vi "Undo.vi"(8 "error in (no error)":errorcluster, 11 "All Queue in":T2) -> (0 "error out":errorcluster, 2 "Ctrl Val.Get All":T1[](array[typedef]), 3 "All Queue out":T2, 4 "Redo Enable":bool, 6 "Undo Enable":bool)   [LabVIEW 2015, in "UndoLibrary.lvlib"]
doc: "This VI stores the values to perform the undo action."
uses:
  UndoLibrary.lvlib
  Controls/cluster_All Queue.ctl
  Controls/cluster_Control Value.ctl
  QueueOperations/QueueOperations.lvlib
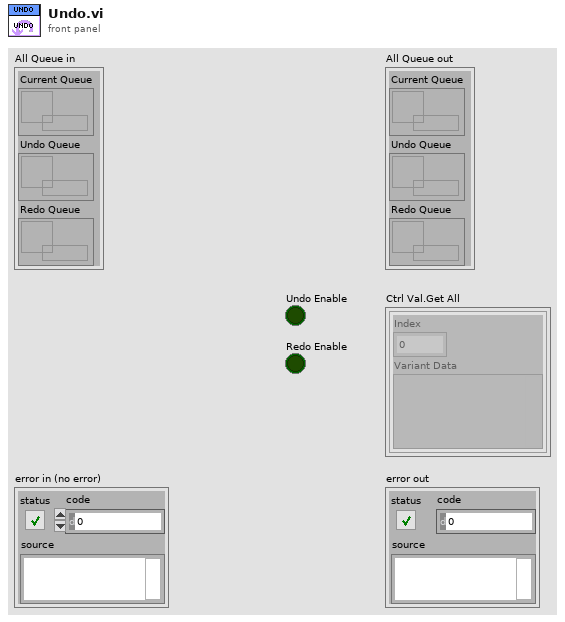
[diagram p1: front panel]
types:
  T1 = typedef "UndoLibrary.lvlib/cluster_Control Value.ctl" = cluster{"Index":i32, "Variant Data":variant}
  T2 = typedef "UndoLibrary.lvlib/cluster_All Queue.ctl" = cluster{"Current Queue":refnum<queue>, "Undo Queue":refnum<queue>, "Redo Queue":refnum<queue>}
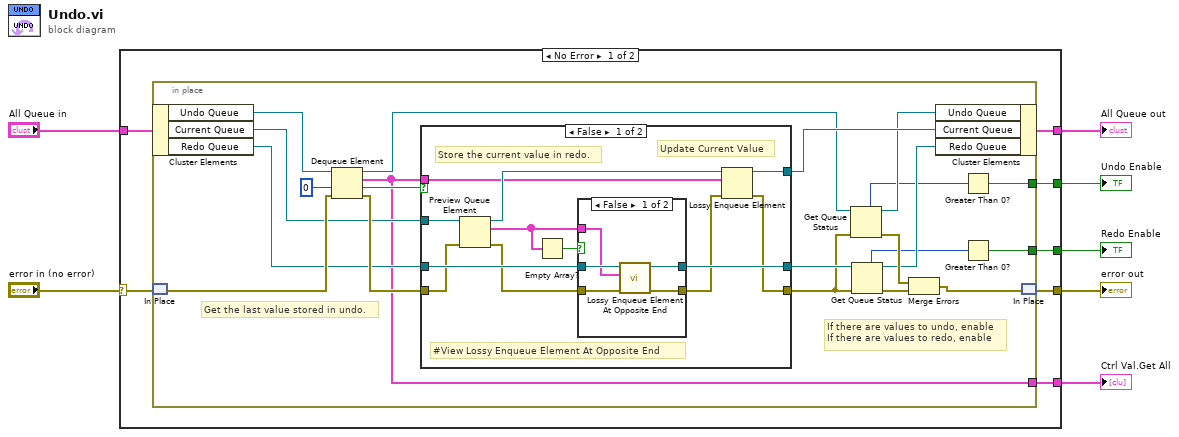
[diagram p0: block diagram]
diagram:
  n1 = case shown="No Error" "error in (no error)" {
    selector: "error in (no error)" -> [w14 w59]
    tunnel: [w13 w59] -> w7
    tunnel: "All Queue in" -> [w12 w58]
    tunnel: [w11 w58] -> w4
    tunnel: [w10 _] -> w3
    tunnel: [w9 _] -> w2
    tunnel: [w8 _] -> w1
    frame No Error {
      n2 = in-place {
        in-place-border: [w28] -> w10
        in-place-border: [w17] -> w9
        in-place-border: [w15] -> w8
        # "Get the last value stored in undo."
        # "If there are values to undo, enable\nIf there are values to redo, enable"
        n3 = in-place-cluster #1(w12) -> ("Undo Queue"=w31:refnum<queue>, "Current Queue"=w30:refnum<queue>, "Redo Queue"=w29:refnum<queue>)
        n4 = in-place-match #2(w14) -> (w32:errorcluster)
        n5 = Dequeue Element(queue=w31, timeout in ms (-1)=0, error in (no error)=w32) -> (queue out=w21:refnum<queue>, element=w28:T1[], timed out?=w35:bool, error out=w33:errorcluster)
        n6 = case shown="False" w35 {
          tunnel: w29 -> [w46 w57]
          tunnel: [w45 w57] -> w27
          tunnel: w28 -> [w38 _]
          tunnel: w30 -> [w44 w56]
          tunnel: w33 -> [w43 w55]
          tunnel: [w39 w56] -> w26
          tunnel: [w41 w55] -> w24
          frame False {
            # "Store the current value in redo."
            # "Update Current Value"
            # "#View Lossy Enqueue Element At Opposite End"
            n7 = Preview Queue Element(queue=w44, error in (no error)=w43) -> (queue out=w40:refnum<queue>, element=w42:T1[], error out=w37:errorcluster)  [unwired: 1 in, 1 out]
            n8 = Empty Array?(array=w42) -> (empty?=w47:bool)
            n9 = case shown="False" w47 {
              tunnel: w37 -> [w50 w53]
              tunnel: w46 -> [w52 w54]
              tunnel: [w49 w54] -> w45
              tunnel: [w48 w53] -> w36
              tunnel: w42 -> [w51 _]
              frame False {
                n10 = call "Lossy Enqueue Element At Opposite End.vi"("error in (no error)"=w50, "element"=w51, "queue in"=w52) -> ("error out"=w48:errorcluster, "queue out"=w49:refnum<queue>)  [unwired: 5 in, 2 out]
              }
              frame True {
              }
            }
            n11 = Lossy Enqueue Element(queue=w40, element=w38, error in (no error)=w36) -> (queue out=w39:refnum<queue>, error out=w41:errorcluster)  [unwired: 2 out]
          }
          frame True {
          }
        }
        n12 = Get Queue Status(queue=w21, error in (no error)=w24) -> (queue out=w20:refnum<queue>, error out=w22:errorcluster, # elements in queue=w18:i32)  [unwired: 1 in, 5 out]
        n13 = Get Queue Status(queue=w27, error in (no error)=w24) -> (queue out=w19:refnum<queue>, error out=w25:errorcluster, # elements in queue=w16:i32)  [unwired: 1 in, 5 out]
        n14 = Merge Errors(w22, w25) -> (w23:errorcluster)
        n15 = in-place-cluster #1("Undo Queue"=w20, "Current Queue"=w26, "Redo Queue"=w19) -> (w11:T2)
        n16 = Greater Than 0?(x=w18) -> (x > 0?=w17:bool)
        n17 = Greater Than 0?(x=w16) -> (x > 0?=w15:bool)
        n18 = in-place-match #2(w23) -> (w13:errorcluster)
      }
    }
    frame Error {
    }
  }
  "error out" <- w7
  "All Queue out" <- w4
  "Ctrl Val.Get All" <- w3
  "Undo Enable" <- w2
  "Redo Enable" <- w1
